vi "deserialize.ob.cmd.vi"(11 "DataIn":u64[](array[numeric]) format="%.0x") -> (3 "OrderBook.Command[]":T1[](array[typedef]))   [LabVIEW 2020, in "fpganow.common.host.lvlib"]
uses:
  fpganow.common.host.lvlib
  fpga/orderbook.command.ctl
  fpga/orderbook.command.type.ctl
  fpga/fpganow.common.fpga.lvlib
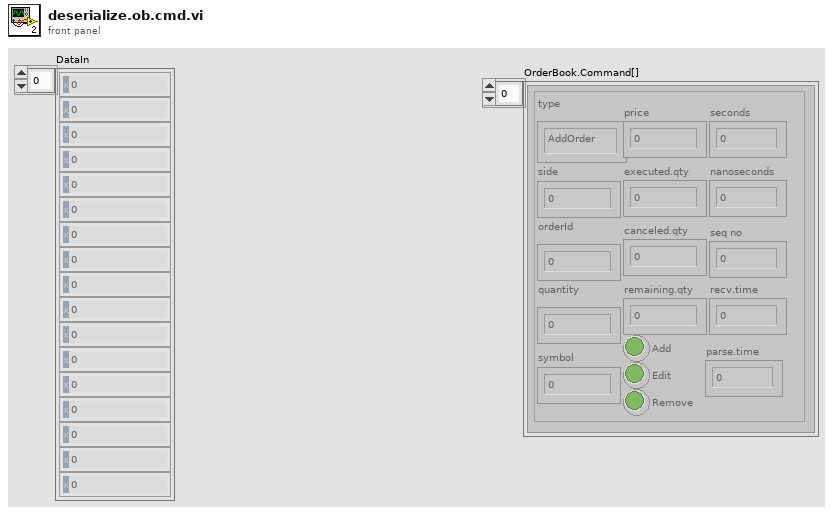
[diagram p1: front panel]
types:
  T1 = typedef "fpganow.common.fpga.lvlib/orderbook.command.ctl" = cluster{"type":T2, "side":u8, "orderId ":u64, "quantity":u32, "symbol":u64, "price":u64, "executed.qty":u32, "canceled.qty":u32, "remaining.qty":u32, "seconds":u64, "nanoseconds":u64, "Add":bool, "Edit":bool, "Remove":bool, "seq no":u32, "recv.time":u64, "parse.time":u64}
  T2 = typedef "fpganow.common.fpga.lvlib/orderbook.command.type.ctl" = enum8{"Time", "AddOrder", "OrderExecuted", "OrderExecutedAtPrice", "ReduceSize", "ModifyOrder", "DeleteOrder", "Get.Everything", "Get.All.Orders", "Get.Top"}
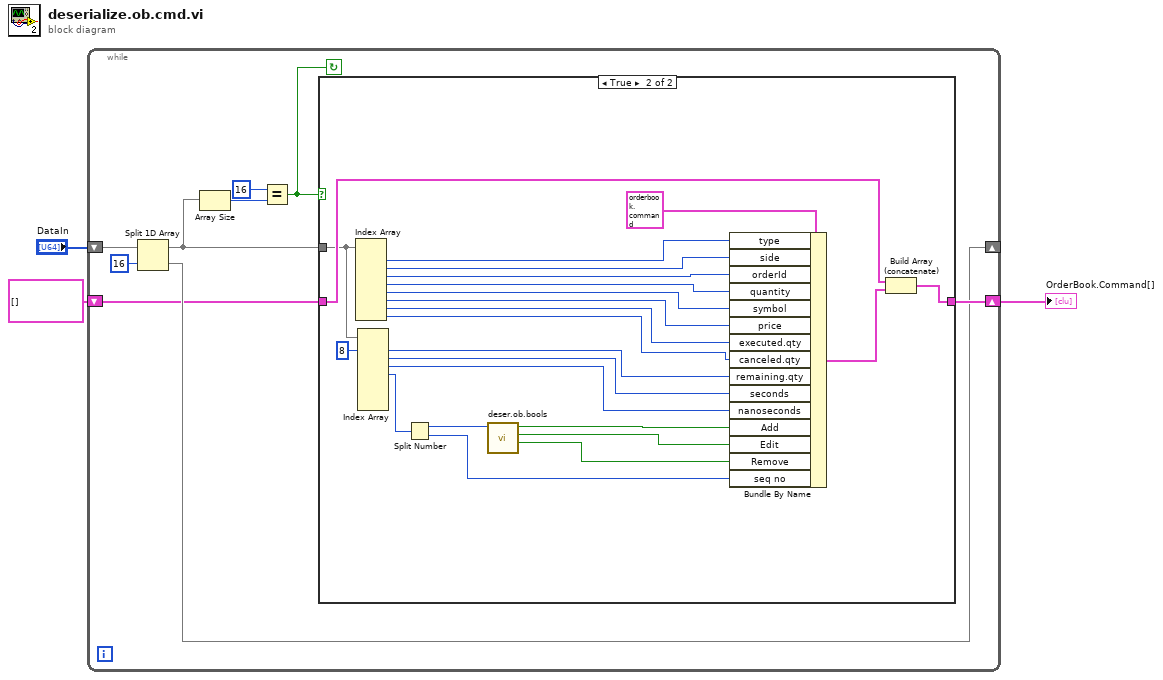
[diagram p0: block diagram]
diagram:
  n1 = while {
    shift-right: [w8] -> _
    shift-left: "DataIn" -> [w12]
    shift-right: [w10] -> w2
    shift-left: T1[] [] -> [w4]
    stop <- w5 continue-if-true
    n2 = Split 1D Array(array=w12, index=16) -> (first subarray=w9:u64[], second subarray=w8:u64[])
    n3 = Array Size(array=w9) -> (size(s)=w7:i32)
    n4 = Equal?(x=16, y=w7) -> (x = y?=w5:bool)
    n5 = case shown="True" w5 {
      tunnel: [w13 w26] -> w10
      tunnel: w9 -> [_ w24]
      tunnel: w4 -> [w13 w25]
      frame False {
      }
      frame True {
        n6 = Index Array(array=w24) -> (element #1=w35:u64, element #2=w34:u64, element #3=w33:u64, element #4=w32:u64, element #5=w31:u64, element #6=w30:u64, element #7=w29:u64, element #8=w28:u64)  [unwired: 8 in]
        n7 = Index Array(array=w24, index #1=8 ("index")) -> (element #1=w22:u64, element #2=w21:u64, element #3=w20:u64, element #4=w19:u64)  [unwired: 7 in, 4 out]
        n8 = Split Number(x=w19) -> (hi(x)=w17:u32, lo(x)=w18:u32)
        n9 = call "deser.ob.bools.vi"("Numeric"=w17) -> ("Remove"=w14:bool, "Edit"=w15:bool, "Add"=w16:bool)  [unwired: 8 in]
        n10 = Bundle By Name(cluster=T1 {"type"=enum."AddOrder", "side"=0, "orderId "=0, "quantity"=0, "symbol"=0, "price"=0, "executed.qty"=0, "canceled.qty"=0, "remaining.qty"=0, "seconds"=0, "nanoseconds"=0, "Add"=FALSE, "Edit"=FALSE, "Remove"=FALSE, "seq no"=0, "recv.time"=0, "parse.time"=0} ("Cluster"), "type"=w35, "side"=w34, "orderId"=w33, "quantity"=w32, "symbol"=w31, "price"=w30, "executed.qty"=w29, "canceled.qty"=w28, "remaining.qty"=w22, "seconds"=w21, "nanoseconds"=w20, "Add"=w16, "Edit"=w15, "Remove"=w14, "seq no"=w18) -> (w27:T1)
        n11 = Build Array (concatenate)(w25, w27) -> (w26:T1[])
      }
    }
  }
  "OrderBook.Command[]" <- w2
